vi "read bpm.vi"() -> ()   [LabVIEW 2009]
uses:
  <vilib>/eio/EIONode/EIONode.xnode
  <vilib>/rvi/eio/nirviEIOImplementation/nirviEIOImplementation.xnode
  <vilib>/rvi/eio/common/nirviEmuTemplateMethod_errors.vi
  <vilib>/rvi/eio/common/nirviEmuClasses.ctl
  <vilib>/rvi/eio/nirviErrorMerge/nirviErrorMerge.xnode
  <vilib>/rvi/eio/common/nirviEmuTemplateMethod_noerrors.vi
panel:
  out "trigger":fxp<+/-,26,5>[](array[numeric]) format="%.23g"
  out "signal":fxp<+/-,26,5>[](array[numeric]) format="%.23g"
  out "Trig Edge":bool
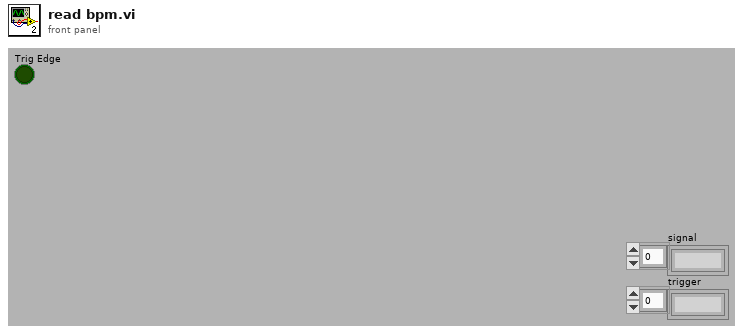
[diagram p1: front panel]
types:
  T1 = typedef "nirviEmuClasses.ctl" = enum16{"IO Read", "IO Write", "Method", "Property Read", "Property Write"}
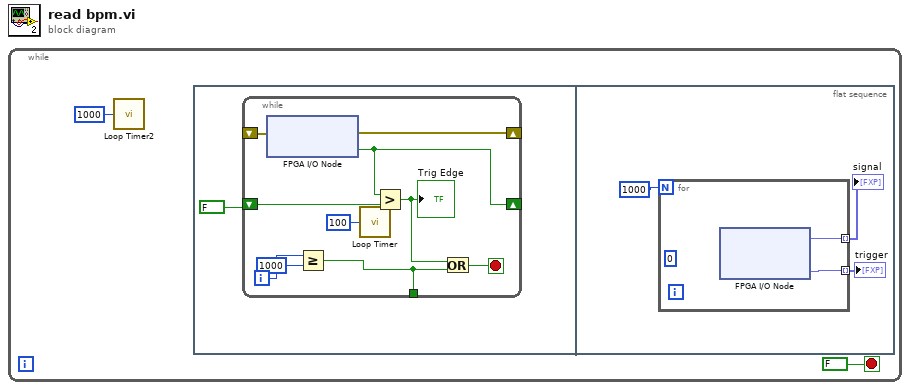
[diagram p0: block diagram]
diagram:
  n1 = while {
    stop <- FALSE stop-if-true
    n2 = call "Loop Timer2"("Count(uSec)"=u32 1000) -> ()  [unwired: 1 out]
    n3 = flat-sequence {
      frame #0 {
        n4 = while {
          shift-right: [w12] -> _
          shift-left: FALSE ("Trig Edge 2") -> [w13]
          tunnel: [w5] -> _
          shift-right: [w8] -> _
          shift-left: _ -> [w9]
          i -> [w6]
          stop <- w11 stop-if-true
          n5 = xnode "FPGA I/O Node"("error in"=w9) -> ("error out"=w8:errorcluster, "Mod2/Trig"=w12:bool)  [unwired: 1 in, 1 out]
          n6 = Greater Or Equal?(x=w6, y=1000) -> (x >= y?=w5:bool)
          n7 = call "Loop Timer"("Count(uSec)"=u32 100) -> ()  [unwired: 1 out]
          n8 = Greater?(x=w12, y=w13) -> (0:w10:bool)
          "Trig Edge" <- w10
          n9 = Or(x=w10, y=w5) -> (x .or. y?=w11:bool)
        }
      }
      frame #1 {
        n10 = for {
          N: 1000 -> [_]
          tunnel: [w76] -> w73 mode=indexing
          tunnel: [w75] -> w74 mode=indexing
          (unwired) u16 0 ("Configuration [i+2]")
          n11 = xnode "FPGA I/O Node"() -> ("Mod2/AI0"=w75:fxp<+/-,26,5>, "Mod2/AI1"=w76:fxp<+/-,26,5>)  [unwired: 2 in, 2 out]
        }
        "signal" <- w74
        "trigger" <- w73
      }
    }
  }
